vi "arraydouble.vi"(2 "Array In":dbl[](array[numeric]) format="%.2f", 3 "Base":dbl format="%.2f") -> (0 "Array Out (not in place)":dbl[](array[numeric]) format="%0.2f", 1 "Array Out":dbl[](array[numeric]) format="%.2f")   [LabVIEW 2011]
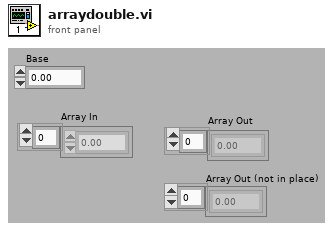
[diagram p1: front panel]
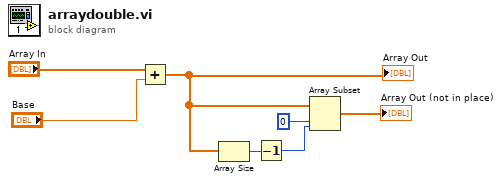
[diagram p0: block diagram]
diagram:
  n1 = Add(x="Array In", y="Base") -> (x+y=w5:dbl[])
  "Array Out" <- w5
  n2 = Array Size(array=w5) -> (size(s)=w2:i32)
  n3 = Decrement(x=w2) -> (x-1=w3:i32)
  n4 = Array Subset(array=w5, index=0, length=w3) -> (→"Array Out (not in place)":dbl[])
